vi "InsertNewValue.vi"(11 "Board":i32[][](array[numeric])=[[0, 0, 0, 0], [0, 0, 0, 0], [0, 0, 0, 0], [0, 0, 0, 0]]) -> (3 "output":i32[][](array[numeric]))   [LabVIEW 2010]
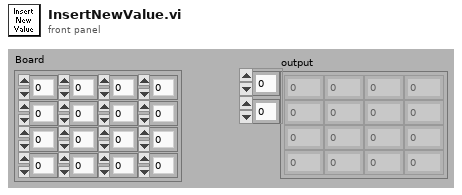
[diagram p1: front panel]
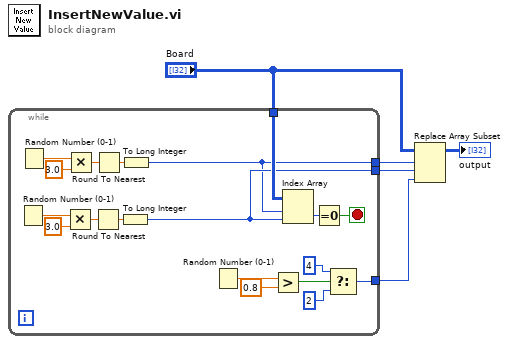
[diagram p0: block diagram]
diagram:
  n1 = while {
    tunnel: [w12] -> w5
    tunnel: [w13] -> w4
    tunnel: "Board" -> [w20]
    tunnel: [w6] -> w1
    stop <- w18 stop-if-true
    n2 = Random Number (0-1)() -> (number: 0 to 1=w14:dbl)
    n3 = Random Number (0-1)() -> (number: 0 to 1=w24:dbl)
    n4 = Multiply(x=w14, y=3.0) -> (x*y=w16:dbl)
    n5 = Multiply(x=w24, y=3.0) -> (x*y=w22:dbl)
    n6 = Round To Nearest(number=w16) -> (nearest integer value=w17:dbl)
    n7 = Round To Nearest(number=w22) -> (nearest integer value=w21:dbl)
    n8 = To Long Integer(number=w17) -> (32bit integer=w13:i32)
    n9 = To Long Integer(number=w21) -> (32bit integer=w12:i32)
    n10 = Random Number (0-1)() -> (number: 0 to 1=w11:dbl)
    n11 = Greater?(x=w11, y=0.8) -> (0:w8:bool)
    n12 = Index Array(array=w20, index (row)=w12, index (col)=w13) -> (element=w19:i32)
    n13 = Equal To 0?(x=w19) -> (x = 0?=w18:bool)
    n14 = Select(t=4 ("index (row)"), s=w8, f=2 ("index (row)")) -> (s? t:f=w6:i32)
  }
  n15 = Replace Array Subset(array="Board", new element=w1, index (row)=w5, index (col)=w4) -> (→"output":i32[][])
